vi "Fundamental Phase Calibration.vi"(0 "one-cycle fundamental vectors in":T2(array[cluster]), 1 "ranges to calibrate [%]":dbl[](array[numeric]), 5 "phase delays [deg]":dbl[][](array[numeric]), 9 "system info in":refnum<class "EP System Info.lvclass">, 11 "error in (no error)":errorcluster, 12 "actual ranges [%]":dbl[](array[numeric])) -> (4 "one-cycle fundamental vectors out":T2(array[cluster]), 10 "system info out":refnum<class "EP System Info.lvclass">, 15 "error out":errorcluster)   [LabVIEW 2014, in "NI_EP_Power Quality.lvlib"]
doc: "Calibrates the phase of a fundamental vector based on <B>actual ranges</B>. You can use the Get Range Utilization VI to calculate <B>actual ranges</B>.\n\nThis VI supports measuring single-line and multiple-line systems."
uses:
  <vilib>/addons/Electrical Power/PQ/NI_EP_Power Quality.lvlib
  <vilib>/addons/Electrical Power/PQ/Common/Controls/ep_AI Data Channel.ctl
  <vilib>/addons/Electrical Power/PQ/Common/Classes/System Info/EP System Info.lvclass
  <vilib>/addons/Electrical Power/PQ/Scaling_Calibration/subVIs/ep_Compute Third Current (Vectors).vi
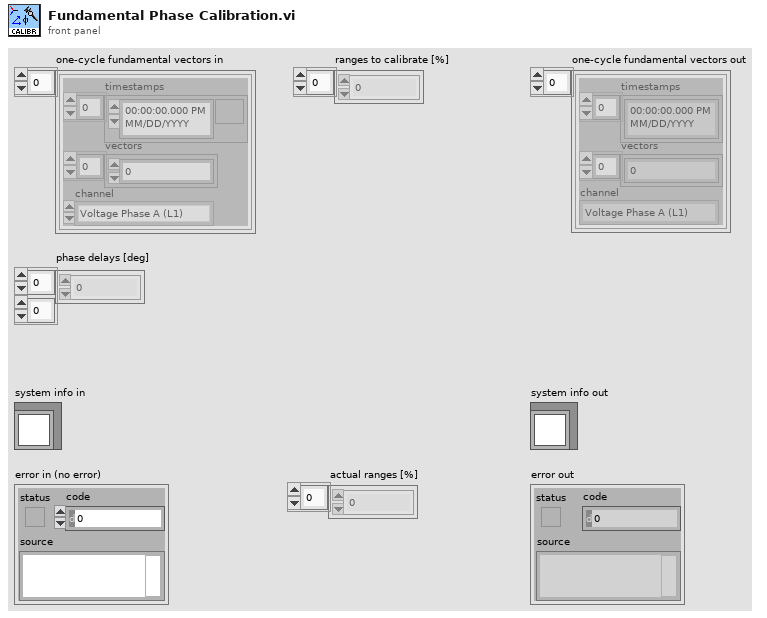
[diagram p1: front panel]
types:
  T1 = typedef "NI_EP_Power Quality.lvlib/ep_AI Data Channel.ctl" = enum16{"Voltage Phase A (L1)", "Voltage Phase B (L2)", "Voltage Phase C (L3)", "Voltage Phase N (Neutral)", "Current Phase A (L1)", "Current Phase B (L2)", "Current Phase C (L3)", "Current Phase N (Neutral)"}
  T2 = cluster{"timestamps":timestamp[], "vectors":cdb[], "channel":T1}[]
  T3 = cluster{"timestamps":timestamp[], "vectors":cdb[], "channel":T1}
  T4 = typedef "NI_EP_Power Quality.lvlib/ep_Wiring.ctl" = enum16{"4xUph + 4xI", "3xUph + 4xI", "3xUline + 4xI", "3xUph + 3xI", "3xUline + 3xI", "3xUph + 2xI", "3xUline + 2xI", "1xUph + 1xI"}
  T5 = cluster{"times":timestamp[], "vectors":cdb[], "channel":T1}[]
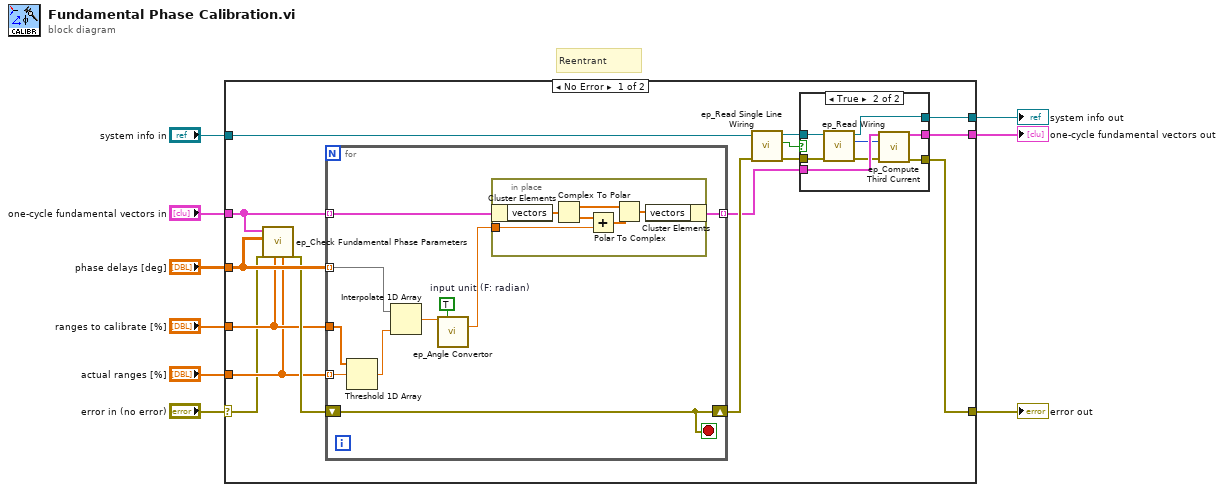
[diagram p0: block diagram]
diagram:
  # "Reentrant"
  n1 = case shown="No Error" "error in (no error)" {
    selector: "error in (no error)" -> [w10 w52]
    tunnel: [w24 w53] -> w9
    tunnel: [w23 w52] -> w8
    tunnel: "one-cycle fundamental vectors in" -> [w22 w53]
    tunnel: "phase delays [deg]" -> [w21 _]
    tunnel: "ranges to calibrate [%]" -> [w19 _]
    tunnel: "actual ranges [%]" -> [w18 _]
    tunnel: "system info in" -> [w17 w54]
    tunnel: [w16 w54] -> w2
    frame No Error {
      n2 = call <vilib>:"ep_Check Fundamental Phase Parameters.vi"("actual ranges [%]"=w18, "ranges to calibrate [%]"=w19, "error in (no error)"=w10, "phase delays [deg]"=w21, "one-cycle fundamental vectors in"=w22) -> ("error out"=w20:errorcluster)  [unwired: 6 in]
      n3 = for {
        tunnel: w22 -> [w44] mode=indexing
        tunnel: w21 -> [w41] mode=indexing
        tunnel: w19 -> [w42]
        tunnel: w18 -> [w45] mode=indexing
        tunnel: [w43] -> w11 mode=indexing
        shift-right: [w36] -> w15
        shift-left: w20 -> [w36]
        stop <- w36 stop-if-true
        w39 = TRUE  # input unit (F: radian)
        n4 = Threshold 1D Array(2:w45, 3:w42) -> (0:w40:dbl)  [unwired: 1 in]
        n5 = Interpolate 1D Array(1:w40, 2:w41) -> (0:w38:dbl)
        n6 = call <vilib>:"ep_Angle Convertor.vi"("input angle"=w38, "input unit (F: radian)"=w39) -> ("angle in radians (-PI..PI)"=w37:dbl)  [unwired: 10 in, 3 out]
        n7 = in-place {
          in-place-border: w37 -> [w47]
          n8 = in-place-cluster #1(w44) -> ("vectors"=w49:cdb[])
          n9 = Complex To Polar(r * e^(i*theta)=w49) -> (r=w51:dbl[], theta=w50:dbl[])
          n10 = Add(x=w50, y=w47) -> (x+y=w46:dbl[])
          n11 = Polar To Complex(1:w46, 2:w51) -> (0:w48:cdb[])
          n12 = in-place-cluster #1("vectors"=w48) -> (w43:T3)
        }
      }
      n13 = call <vilib>:"ep_Read Single Line Wiring.vi"("error in (no error)"=w15, "system info in"=w17) -> ("error out"=w14:errorcluster, "single line wiring? (F)"=w12:bool, "system info out"=w13:refnum<class "EP System Info.lvclass">)  [unwired: 7 in]
      n14 = case shown="True" w12 {
        tunnel: w14 -> [w26 w35]
        tunnel: w13 -> [w25 w34]
        tunnel: w11 -> [w27 w33]
        tunnel: [w27 w30] -> w24
        tunnel: [w26 w29] -> w23
        tunnel: [w25 w28] -> w16
        frame False {
        }
        frame True {
          n15 = call <vilib>:"ep_Read Wiring.vi"("error in (no error)"=w35, "system info in"=w34) -> ("error out"=w32:errorcluster, "wiring"=w31:T4, "system info out"=w28:refnum<class "EP System Info.lvclass">)  [unwired: 6 in, 1 out]
          n16 = call-poly <vilib>:"ep_Compute Third Current.vi"("one period fundamental current vectors in"=w33, "wiring"=w31, "error in (no error)"=w32) -> ("one period fundamental current vectors out"=w30:T5, "error out"=w29:errorcluster)  [unwired: 11 in]
        }
      }
    }
    frame Error {
    }
  }
  "one-cycle fundamental vectors out" <- w9
  "error out" <- w8
  "system info out" <- w2
